vi "CM get machine path.vi"(8 "error in (no error) 2":errorcluster) -> (0 "error in (no error)":errorcluster, 2 "machine path":path)   [LabVIEW 2018]
panel:
  in  "machine path array":string[](array[string])=["C:", "Users", "<empty>", "SPARC4", "COMMAN"]
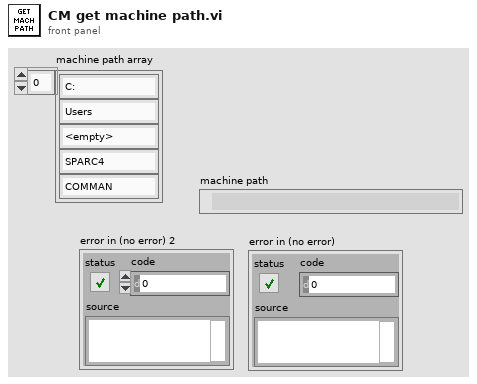
[diagram p1: front panel]
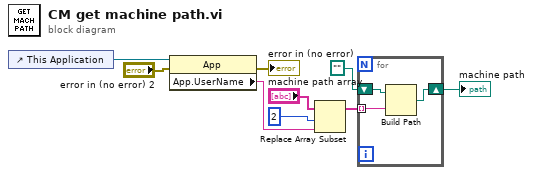
[diagram p0: block diagram]
diagram:
  n1 = control-ref of="This Application"() -> (w9:refnum<vi>)
  n2 = property on="Property Node" class="App"(reference=w9, error in="error in (no error) 2") -> (error out=→"error in (no error)":errorcluster, "App.UserName"=w8:string)  [unwired: 1 out]
  n3 = Replace Array Subset(array="machine path array", new element=w8, index=2) -> (w6:string[])
  n4 = for {
    tunnel: w6 -> [w12] mode=indexing
    shift-right: [w11] -> w4
    shift-left: path "" -> [w10]
    n5 = Build Path(base path=w10, name or relative path=w12) -> (appended path=w11:path)
  }
  "machine path" <- w4
